vi "ArenPID.vi"(4 "Reset?":bool, 6 "Bounds":cluster{"Minimum":dbl, "Maximum":dbl}, 9 "Gains":T1, 10 "Process":dbl, 11 "Setpoint":dbl) -> (3 "Output":dbl)   [LabVIEW 2012]
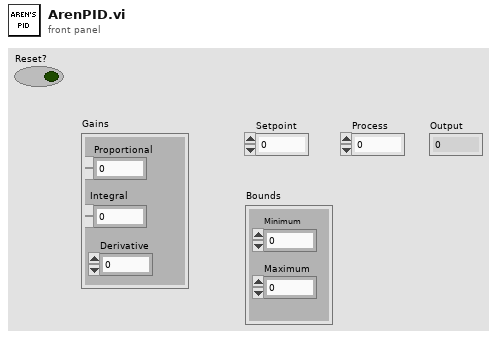
[diagram p1: front panel]
types:
  T1 = cluster{"Proportional":dbl, "Integral":dbl, "Derivative":dbl}
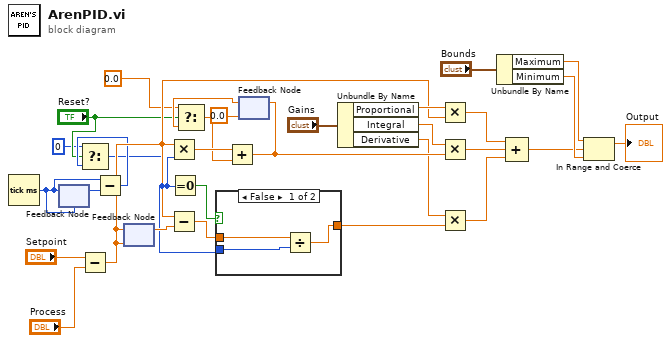
[diagram p0: block diagram]
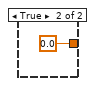
[diagram p2: hidden frame]
diagram:
  n1 = Tick Count (ms)() -> (millisecond timer value=w23:u32)
  n2 = feedback-in #1(w23) -> ()
  n3 = feedback #1(w23) -> (w24:u32)
  n4 = Subtract(x="Setpoint", y="Process") -> (x-y=w20:dbl)
  n5 = Subtract(x=w23, y=w24) -> (x-y=w4:u32)
  n6 = Select(t=u32 0, s="Reset?", f=w4) -> (s? t:f=w3:u32)
  n7 = feedback-in #2(w20) -> ()
  n8 = feedback #2(w20) -> (w21:dbl)
  n9 = Multiply(x=w20, y=w3) -> (x*y=w22:dbl)
  n10 = Subtract(x=w20, y=w21) -> (x-y=w18:dbl)
  n11 = Equal To 0?(x=w3) -> (x = 0?=w19:bool)
  n12 = case shown="False" w19 {
    tunnel: [w32 0.0] -> w16
    tunnel: w18 -> [w34 _]
    tunnel: w3 -> [w33 _]
    frame False {
      n13 = Divide(x=w34, y=w33) -> (x/y=w32:dbl)
    }
    frame True {
    }
  }
  n14 = feedback #3(0.0) -> (w7:dbl)
  n15 = Select(t=0.0, s="Reset?", f=w7) -> (s? t:f=w6:dbl)
  n16 = Add(x=w22, y=w6) -> (x+y=w25:dbl)
  n17 = feedback-in #3(w25) -> ()
  n18 = Unbundle By Name("Gains") -> ("Proportional"=w28:dbl, "Integral"=w26:dbl, "Derivative"=w17:dbl)
  n19 = Multiply(x=w28, y=w20) -> (x*y=w15:dbl)
  n20 = Multiply(x=w26, y=w25) -> (x*y=w14:dbl)
  n21 = Multiply(x=w17, y=w16) -> (x*y=w13:dbl)
  n22 = Unbundle By Name("Bounds") -> ("Maximum"=w11:dbl, "Minimum"=w10:dbl)
  n23 = Compound Arithmetic op=ADD(w15, w14, w13) -> (w9:dbl)
  n24 = In Range and Coerce(upper limit=w11, x=w9, lower limit=w10) -> (coerced(x)=→"Output":dbl)  [unwired: 1 out]
